vi "Fuzzy Compare DBL.vi"(1 "A":dbl format="%_13g", 2 "B":dbl format="%_13g", 4 "Specified Epsilon (NaN=default)":dbl=nan format="%_13g") -> (6 "Fuzzy Equal?":bool)   [LabVIEW 2023, in "NI-568x RF Power Meter.lvlib" / "SG 2250 Path Accessor.lvclass"]
uses:
  SG 2250 Path Accessor.lvclass
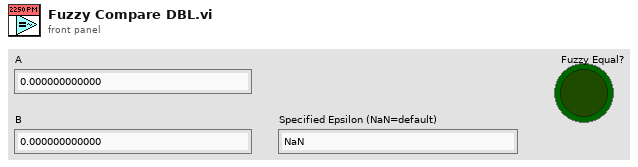
[diagram p1: front panel]
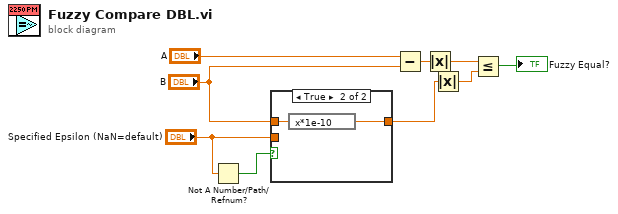
[diagram p0: block diagram]
diagram:
  n1 = Not A Number/Path/Refnum?(number/path/refnum="Specified Epsilon (NaN=default)") -> (NaN/Path/Refnum?=w1:bool)
  n2 = case shown="True" w1 {
    tunnel: [w10 w12] -> w8
    tunnel: "B" -> [_ w11]
    tunnel: "Specified Epsilon (NaN=default)" -> [w10 _]
    frame False {
    }
    frame True {
      n3 = expression code="x*1e-10"(w11) -> (w12:dbl)
    }
  }
  n4 = Subtract(x="A", y="B") -> (x-y=w6:dbl)
  n5 = Absolute Value(x=w6) -> (abs(x)=w7:dbl)
  n6 = Absolute Value(x=w8) -> (abs(x)=w3:dbl)
  n7 = Less Or Equal?(x=w7, y=w3) -> (x <= y?=→"Fuzzy Equal?":bool)
